vi "RobotMain.vi"() -> ()   [LabVIEW 2016]
uses:
  <vilib>/NXT/Subs/LVHSConnector.ctl
  <vilib>/NXT/LegoClasses/BrickReference/BrickReference.lvclass
  <vilib>/NXT/Subs/ColorSensorColors.ctl
  booleanos.ctl
  parametros.ctl
  <vilib>/NXT/Block Support/NXT_InputPort.ctl
  caracteristicas.ctl
  <vilib>/NXT/Block Support/NXT_ButtonSelector.ctl
  <vilib>/NXT/Block Support/NXT_OutputPort.ctl
  <vilib>/NXT/Dual Mode Library/Display/clearDisplay.vi
  <vilib>/NXT/NXTIO Xnodes/NXTIONodeSubVIs/NXTMoveMotors.vi
  <vilib>/NXT/Dual Mode Library/Sensors/readNXTButton.vi
  <vilib>/NXT/NXTIO Xnodes/NXTIONodeSubVIs/NXTStopMotors.vi
  <vilib>/NXT/Dual Mode Library/Waits/Wait_Btn_Press.vi
  <vilib>/NXT/NXTIO Xnodes/AddressXNode/NXTIOAddress.xnode
  <vilib>/NXT/NXTIO Xnodes/NXTIOXNode/NXTIO.xnode
panel:
  out "Boolean 5":bool=TRUE
  out "Boolean 4":bool
  out "Boolean 3":bool
  out "Boolean 2":bool
  out "Boolean":bool
  out "Ang_giroscopio":sgl
  in  "Movimentos \nStop":enum16{"Nada", "Front", "Pega", "Fim"}(ring)
  out "Enable\nreforço SM":bool
  out "Direction Bool":bool
  out "Booleanos e Contadores":T1={"Correct"=FALSE, "Enable State change"=TRUE, "First End"=FALSE, "Intersections crossed"=0.0, "Intersections crossed total"=0.0, "Bonecos"=0.0}
  out "Características":T2={"Colors and Directions"=[enum."Zero", enum."Zero", enum."Zero", enum."Zero", enum."Zero", enum."Zero"], "Direction"=enum."Right", "CS"=enum."Street", "Old Color"=enum."White"}
  in  "Características Iniciais":T2={"Colors and Directions"=[enum."Zero", enum."Zero", enum."Zero", enum."Zero", enum."Zero", enum."Zero"], "Direction"=enum."Right", "CS"=enum."Street", "Old Color"=enum."White"}
  out "Enable 2":bool
  out "Enable":bool
  in  "SC in":bool=TRUE
  in  "CS":T4(ring)
  in  "Parâmetros Iniciais":T5={"Gyro Port"=0, "Sensor - Left"=3, "Sensor - Right"=2, "     Color \nSensor Port"=1, "Kp Front"=0.5, "Motor speed"=-15, "Distance to street"=15.0, "Motor speed turns"=16, "Kp Curvas"=0.3} {"Kp Front" format="%.3f"; "Color \nSensor Port" items=["Port 1", "Port 2", "Port 3", "Port 4"]; "Sensor - Right" items=["Port 1", "Port 2", "Port 3", "Port 4"]; "Sensor - Left" items=["Port 1", "Port 2", "Port 3", "Port 4"]; "Gyro Port" items=["Port 1", "Port 2", "Port 3", "Port 4"]}
  in  "Booleanos e Contadores Iniciais":T1={"Correct"=FALSE, "Enable State change"=TRUE, "First End"=FALSE, "Intersections crossed"=0.0, "Intersections crossed total"=0.0, "Bonecos"=0.0} caption="Booleanos e Contadores"
  out "IdentifyCollor":T3=enum."White"
  out "Collor":T3
  out "NXT/EV3 2":T7
  in  "NXT/EV3":T7
  # "Permite que ocorra troca \nde estados se True e interrompe-as \nse False."
  # "Booleano que retorna F quando chega em Delivery.\nGarantindo que não contará\nmais intersections"
  # "Salva o total de interseções \ncruzadas"
  # "Contador de quantas \ninterseções foram cruzadas.\nSoma ao acertar"
  # "black"
  # "blue"
  # "green"
  # "yellow"
  # "red"
  # "black"
  # "blue"
  # "green"
  # "yellow"
  # "red"
  # "Permite que ocorra troca \nde estados se True e interrompe-as \nse False."
  # "Booleano que retorna F quando chega em Delivery.\nGarantindo que não contará\nmais intersections"
  # "Salva o total de interseções \ncruzadas"
  # "Contador de quantas \ninterseções foram cruzadas.\nSoma ao acertar"
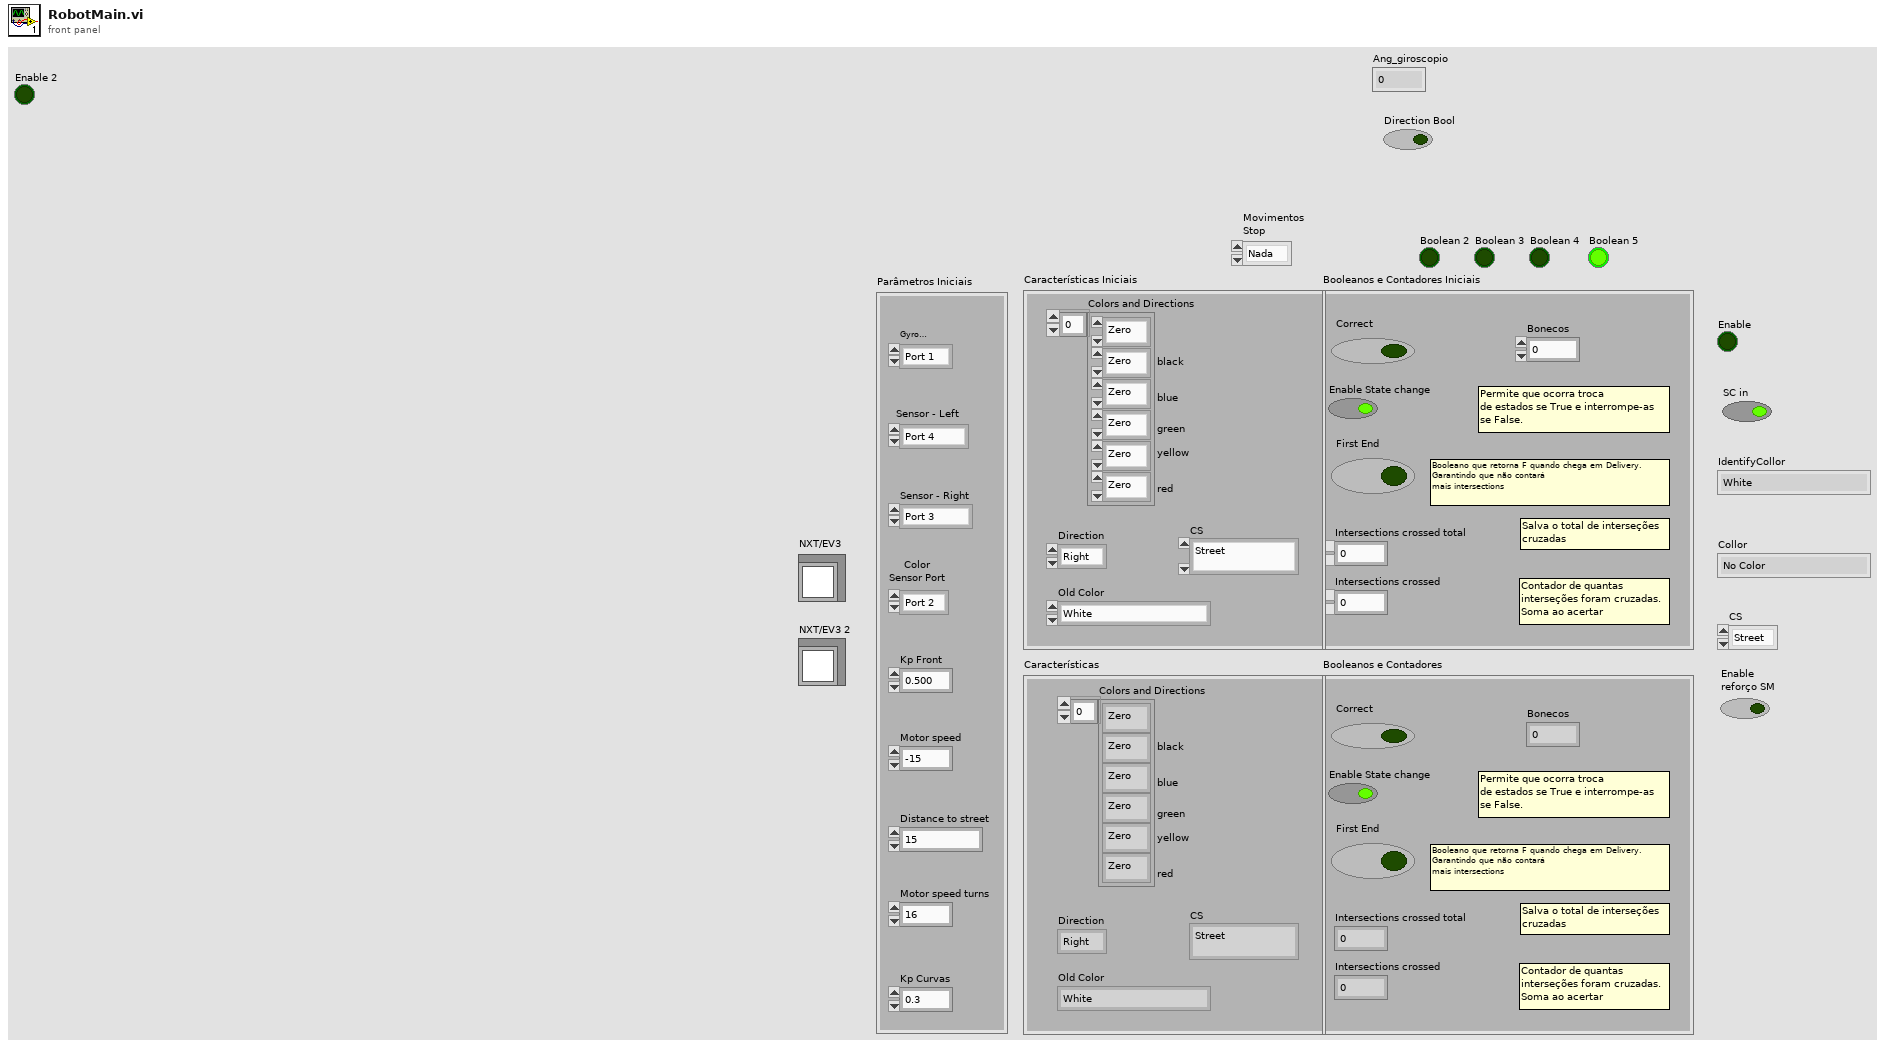
[diagram p1: front panel]
types:
  T1 = typedef "booleanos.ctl" = cluster{"Correct":bool, "Enable State change":bool, "First End":bool, "Intersections crossed":dbl, "Intersections crossed total":dbl, "Bonecos":dbl}
  T2 = typedef "caracteristicas.ctl" = cluster{"Colors and Directions":enum16{"Zero", "Right", "Front", "Left"}[], "Direction":enum16{"Zero", "Right", "Front", "Left"}, "CS":enum16{"Street", "Intersection", "End", "Stop", "Square", "Delivery", "Empty"}, "Old Color":T3}
  T3 = typedef "ColorSensorColors.ctl" = enum16{"No Color", "Black", "Blue", "Green", "Yellow", "Red", "White", "Brown"}
  T4 = enum16{"Street", "Intersection", "End", "Stop", "Square", "Delivery"}
  T5 = typedef "parametros.ctl" = cluster{"Gyro Port":T6, "Sensor - Left":T6, "Sensor - Right":T6, "     Color \nSensor Port":T6, "Kp Front":dbl, "Motor speed":i32, "Distance to street":dbl, "Motor speed turns":i32, "Kp Curvas":dbl}
  T6 = typedef "NXT_InputPort.ctl" = u32
  T7 = typedef "LVHSConnector.ctl" = refnum<class "BrickReference.lvclass">
  T8 = typedef "NXT_OutputPort.ctl" = u8
  T9 = enum16{"Street", "Intersection", "End", "Stop", "Square", "Delivery", "Empty"}
  T10 = typedef "NXT_ButtonSelector.ctl" = u16
  T11 = cluster{"Colors and Directions":enum16{"Zero", "Right", "Front", "Left"}[], "Direction":enum16{"Zero", "Right", "Front", "Left"}, "CS":enum16{"Street", "Intersection", "End", "Stop", "Square", "Delivery"}, "Old Color":T3}
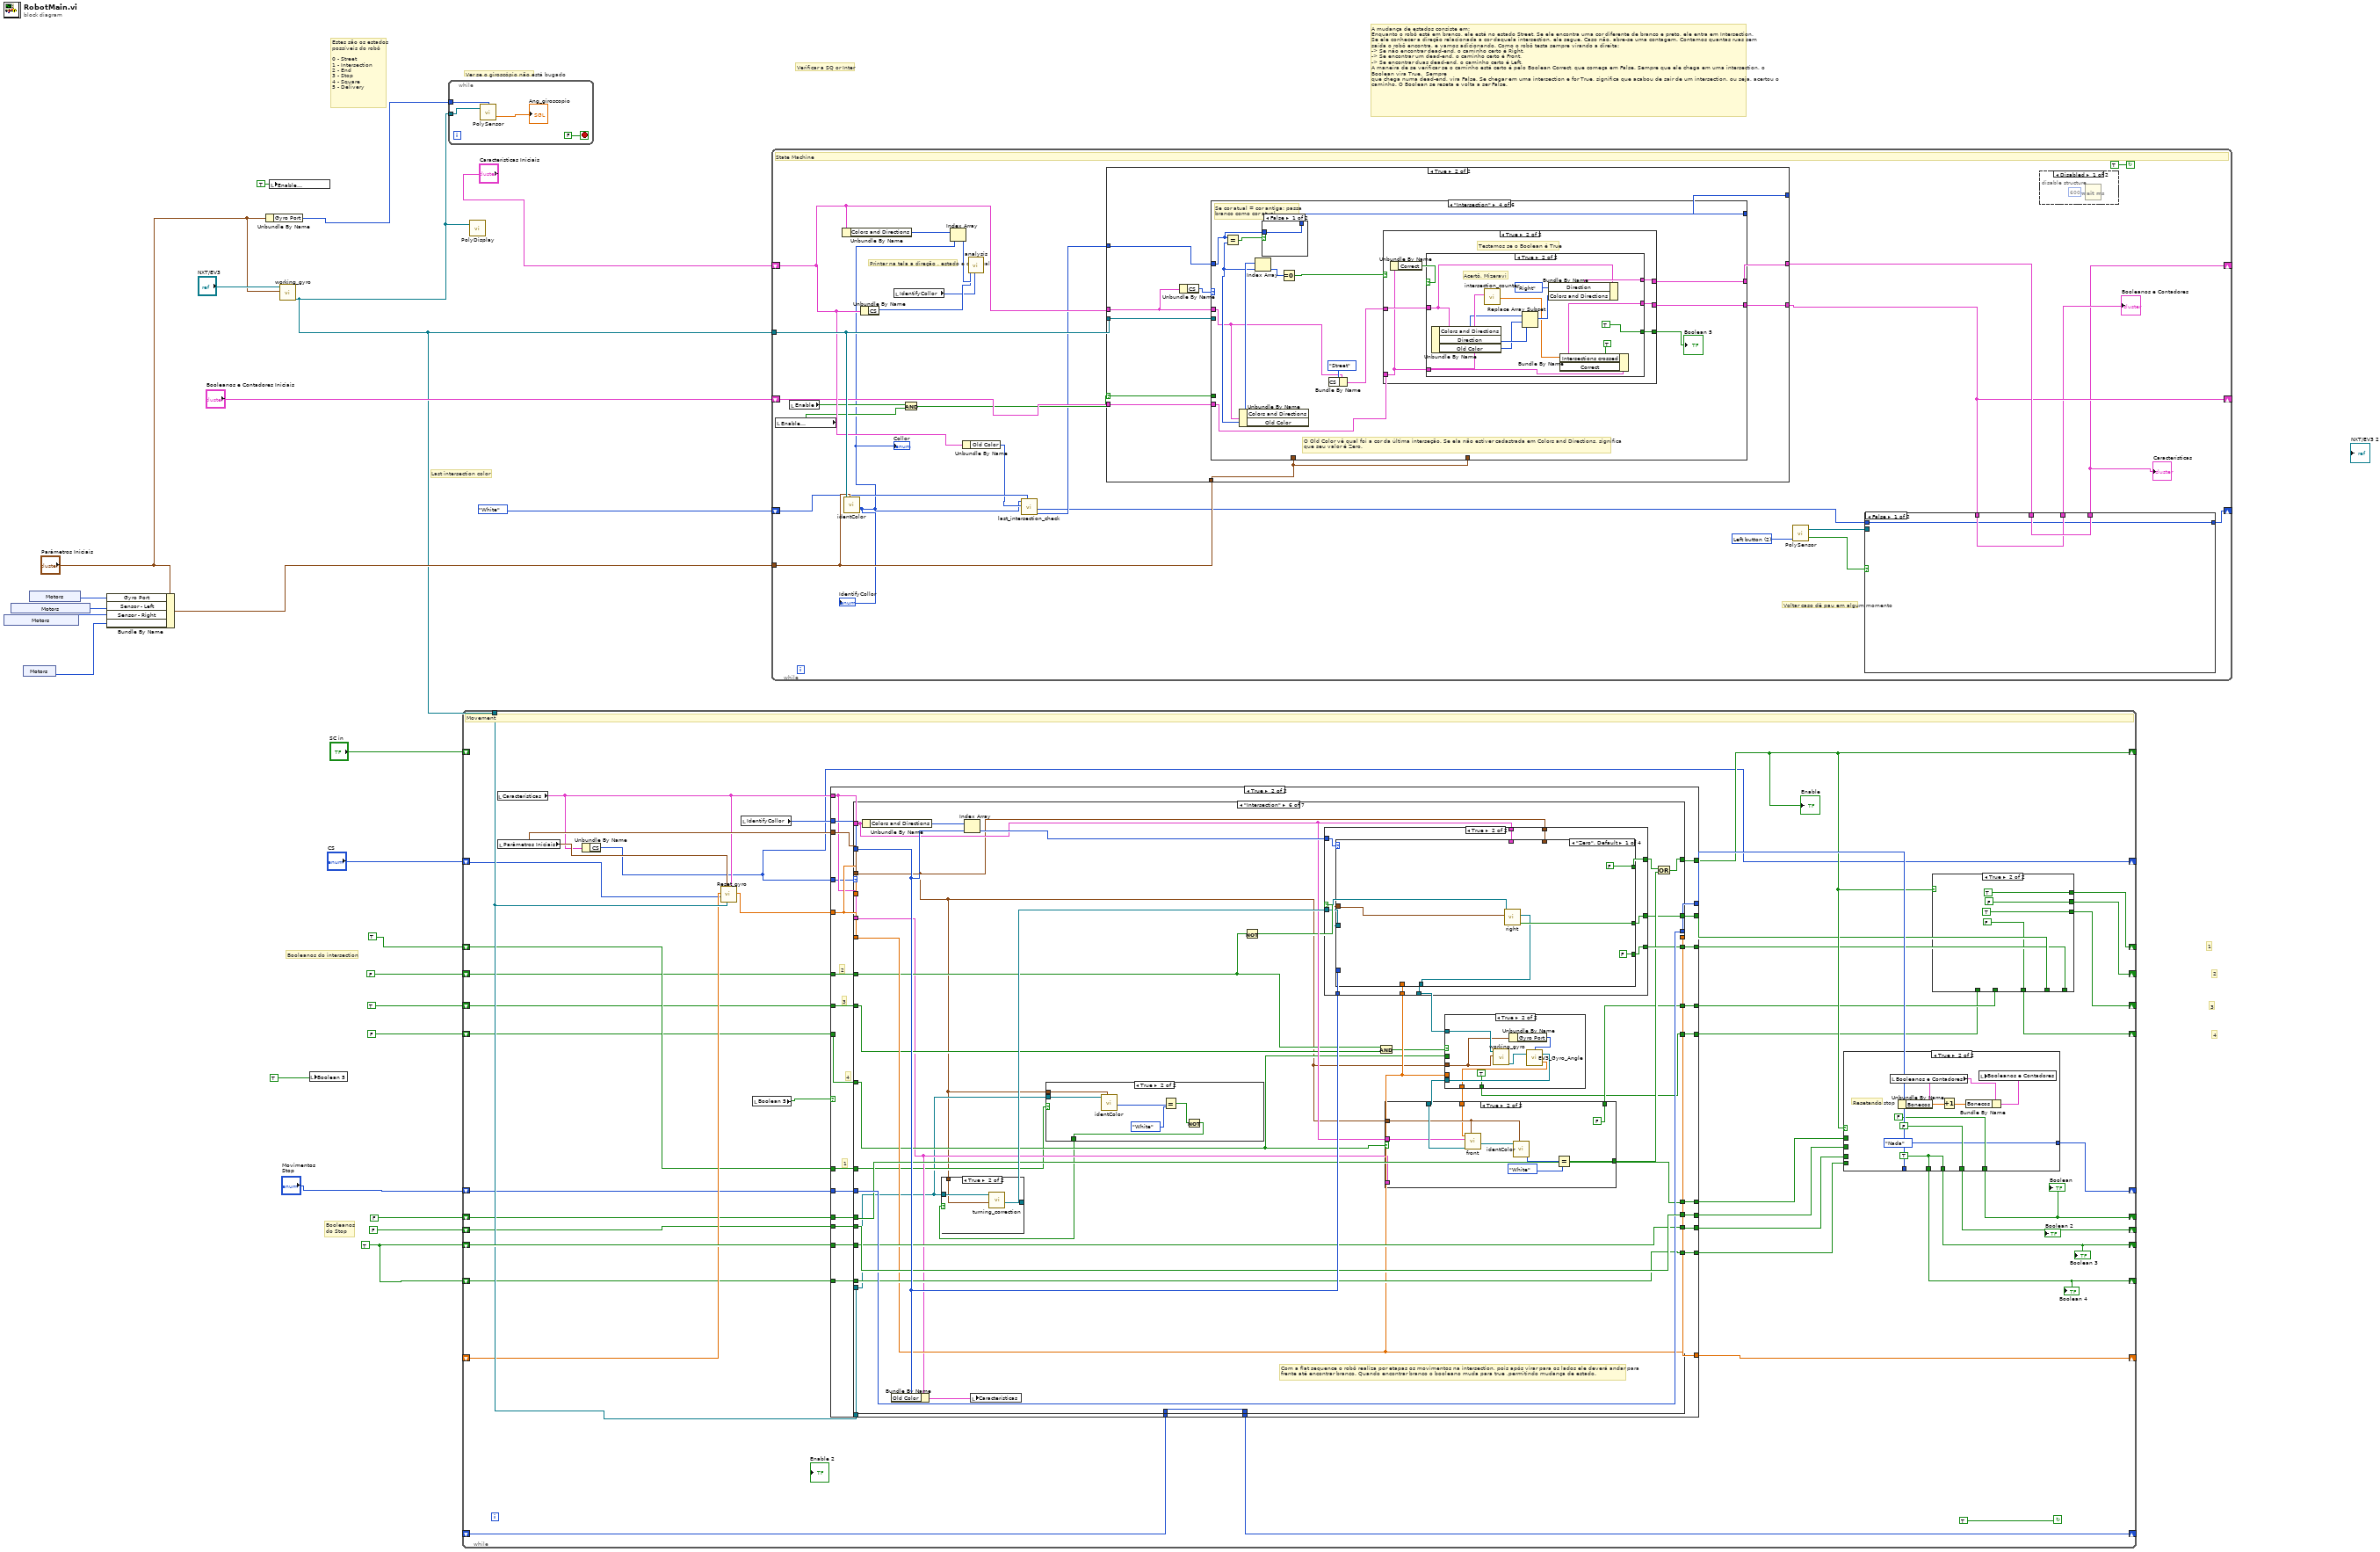
[diagram p0: block diagram]
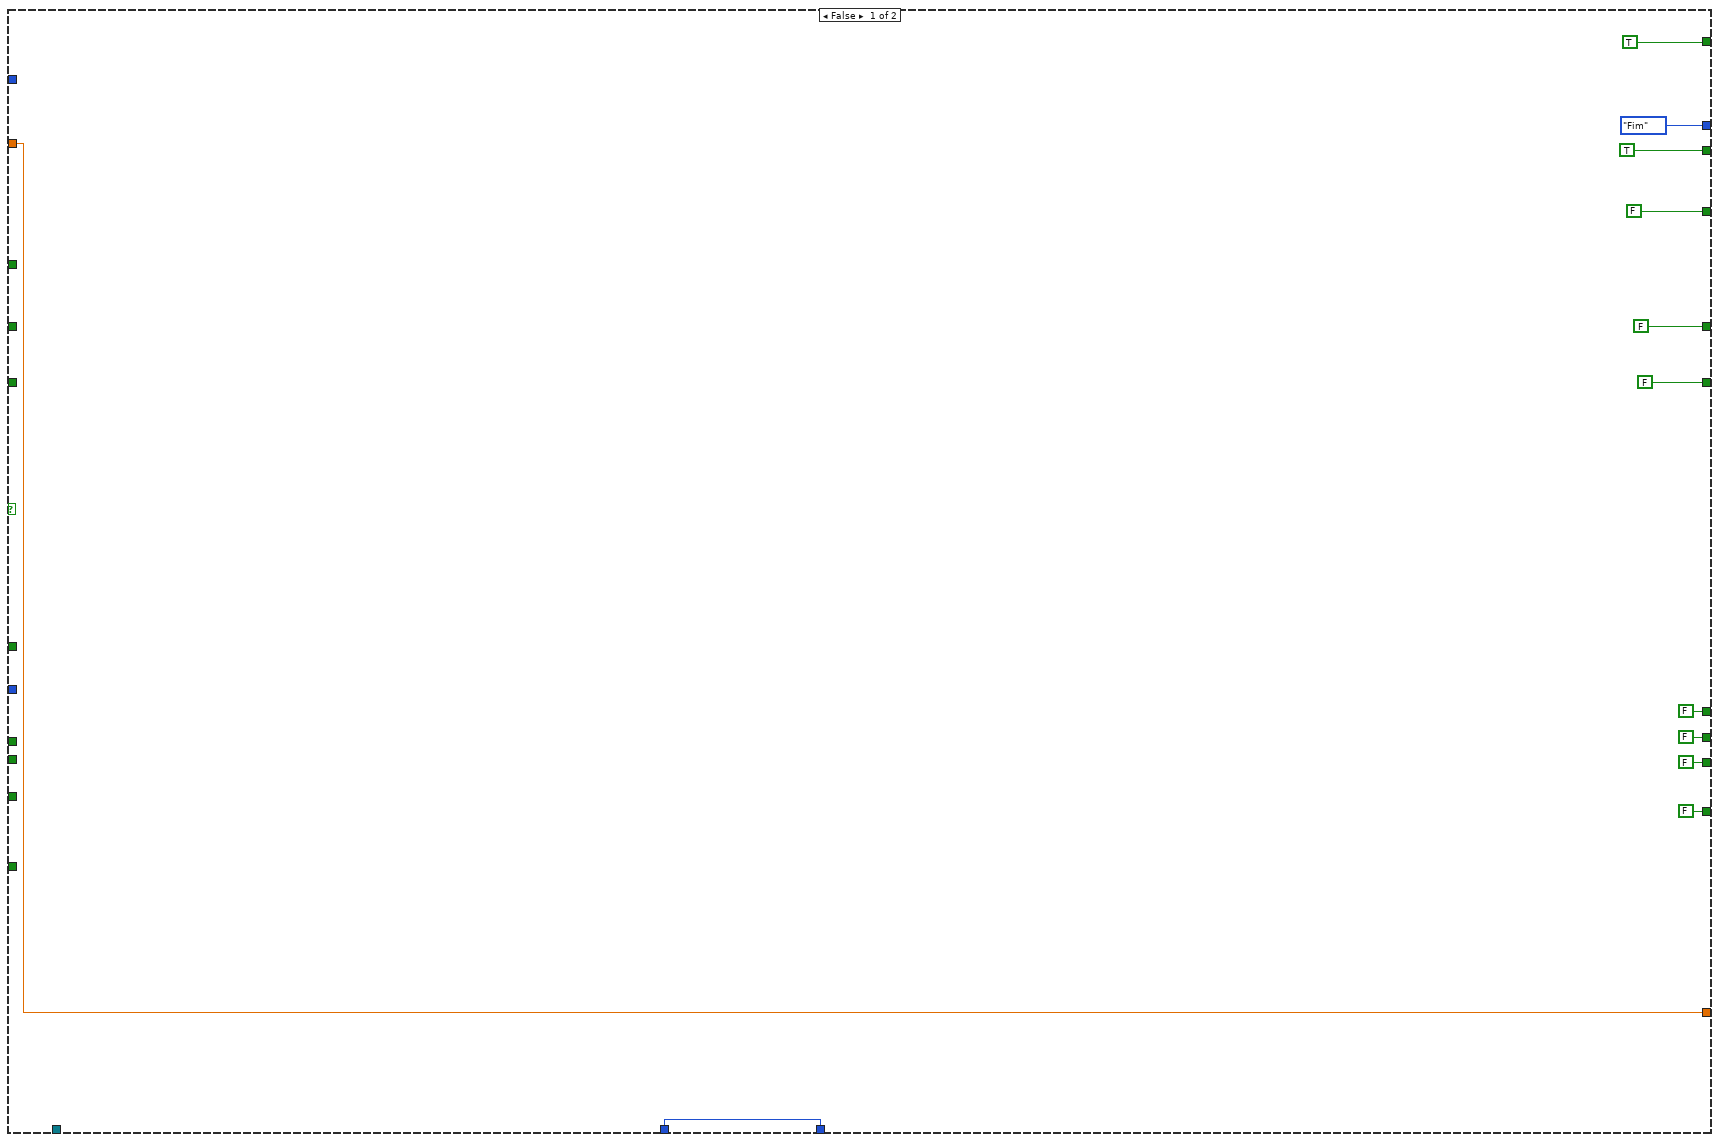
[diagram p2: hidden frame]
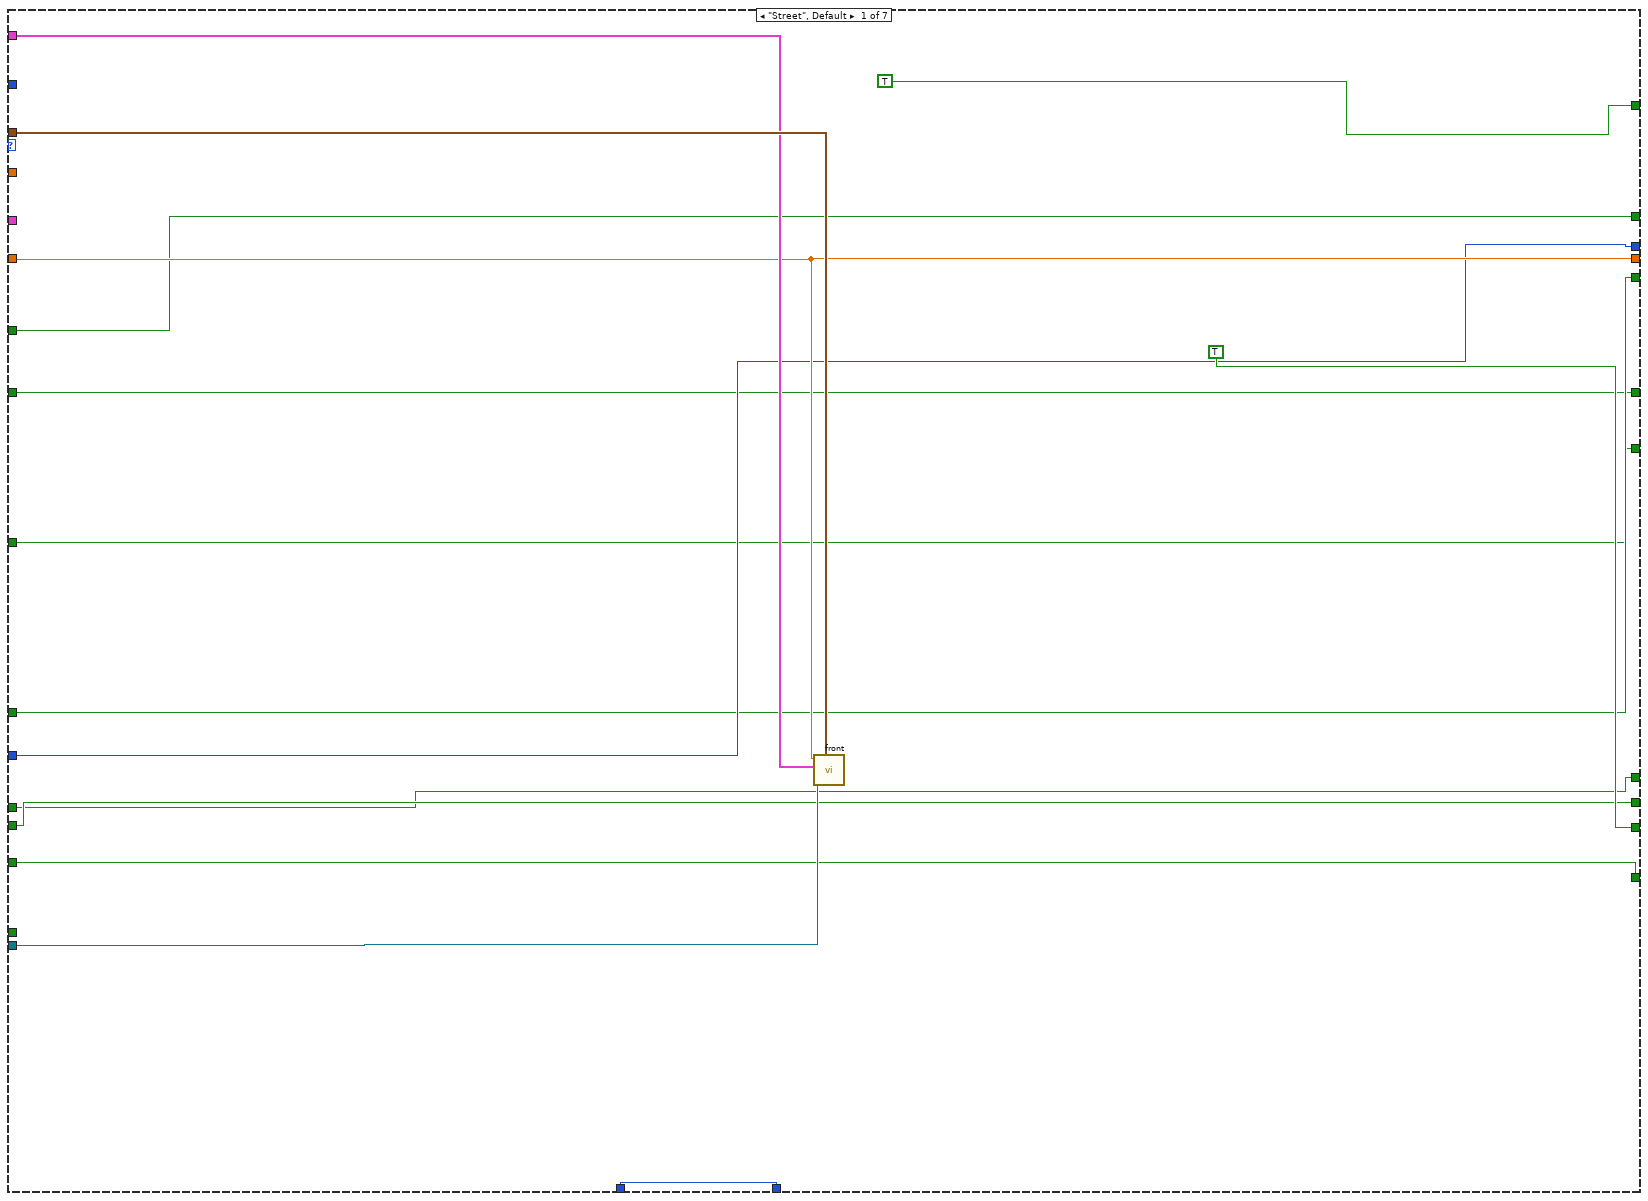
[diagram p3: hidden frame]
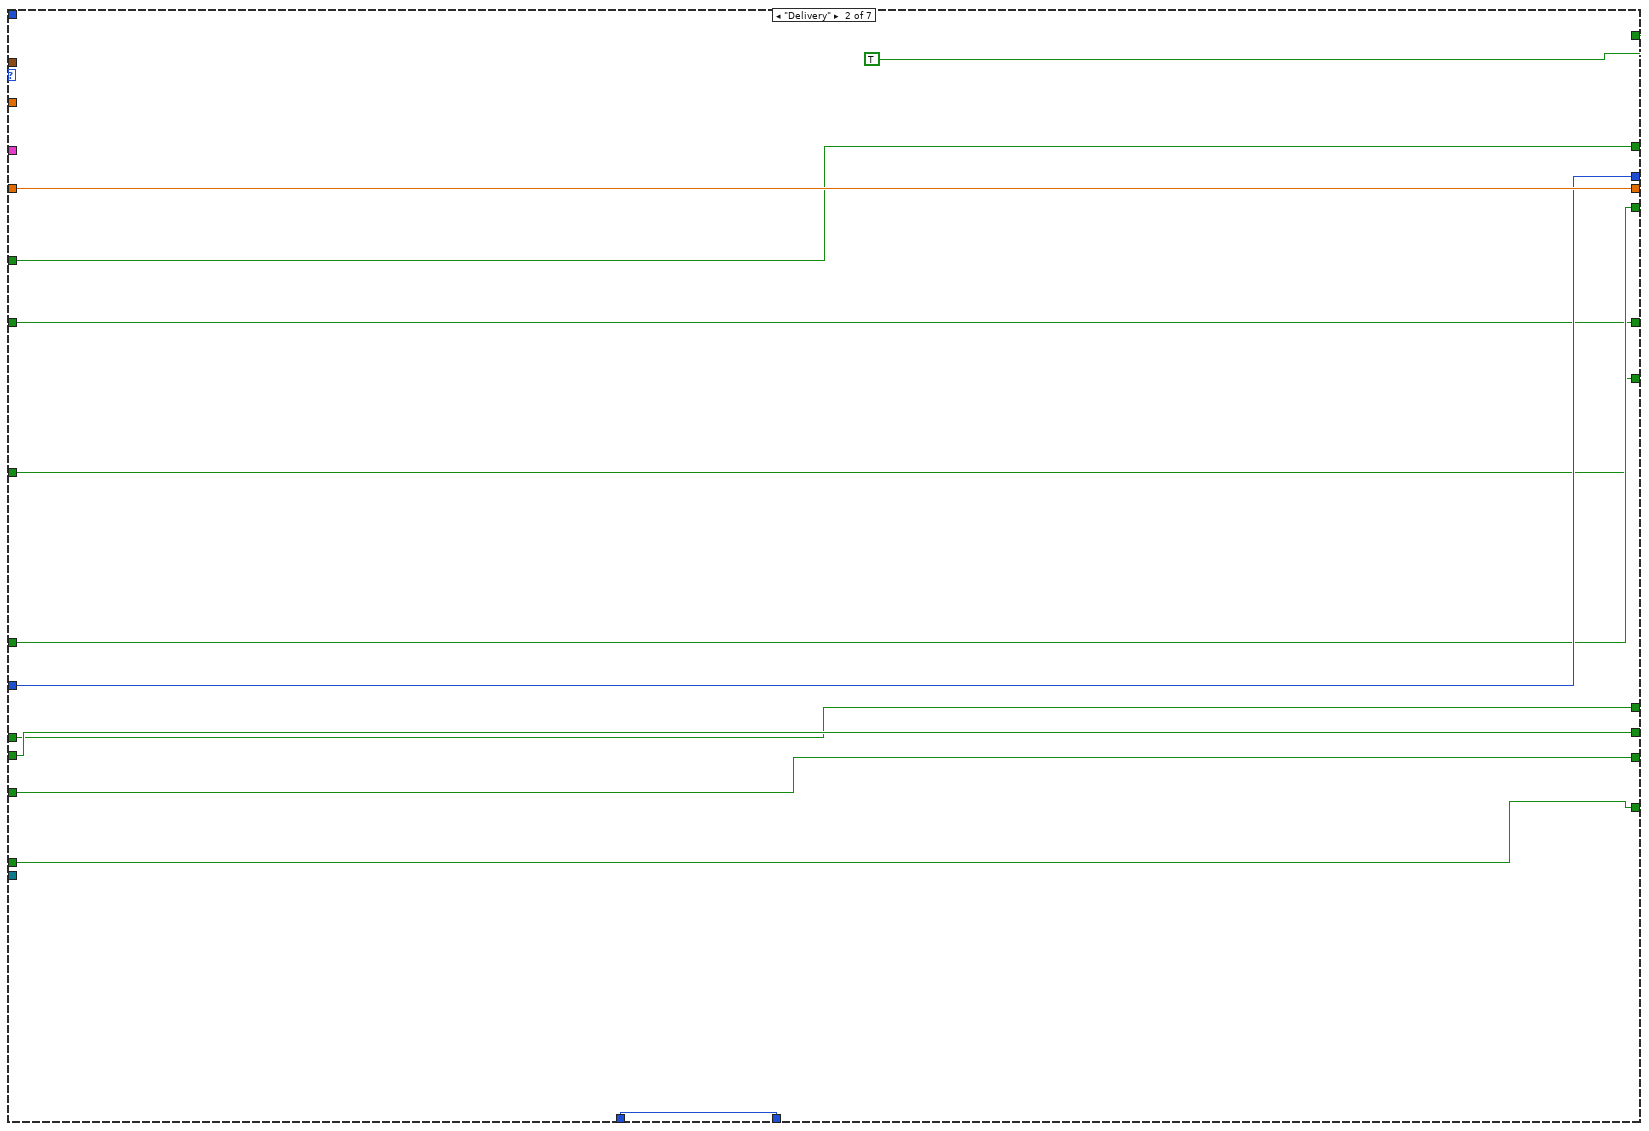
[diagram p4: hidden frame]
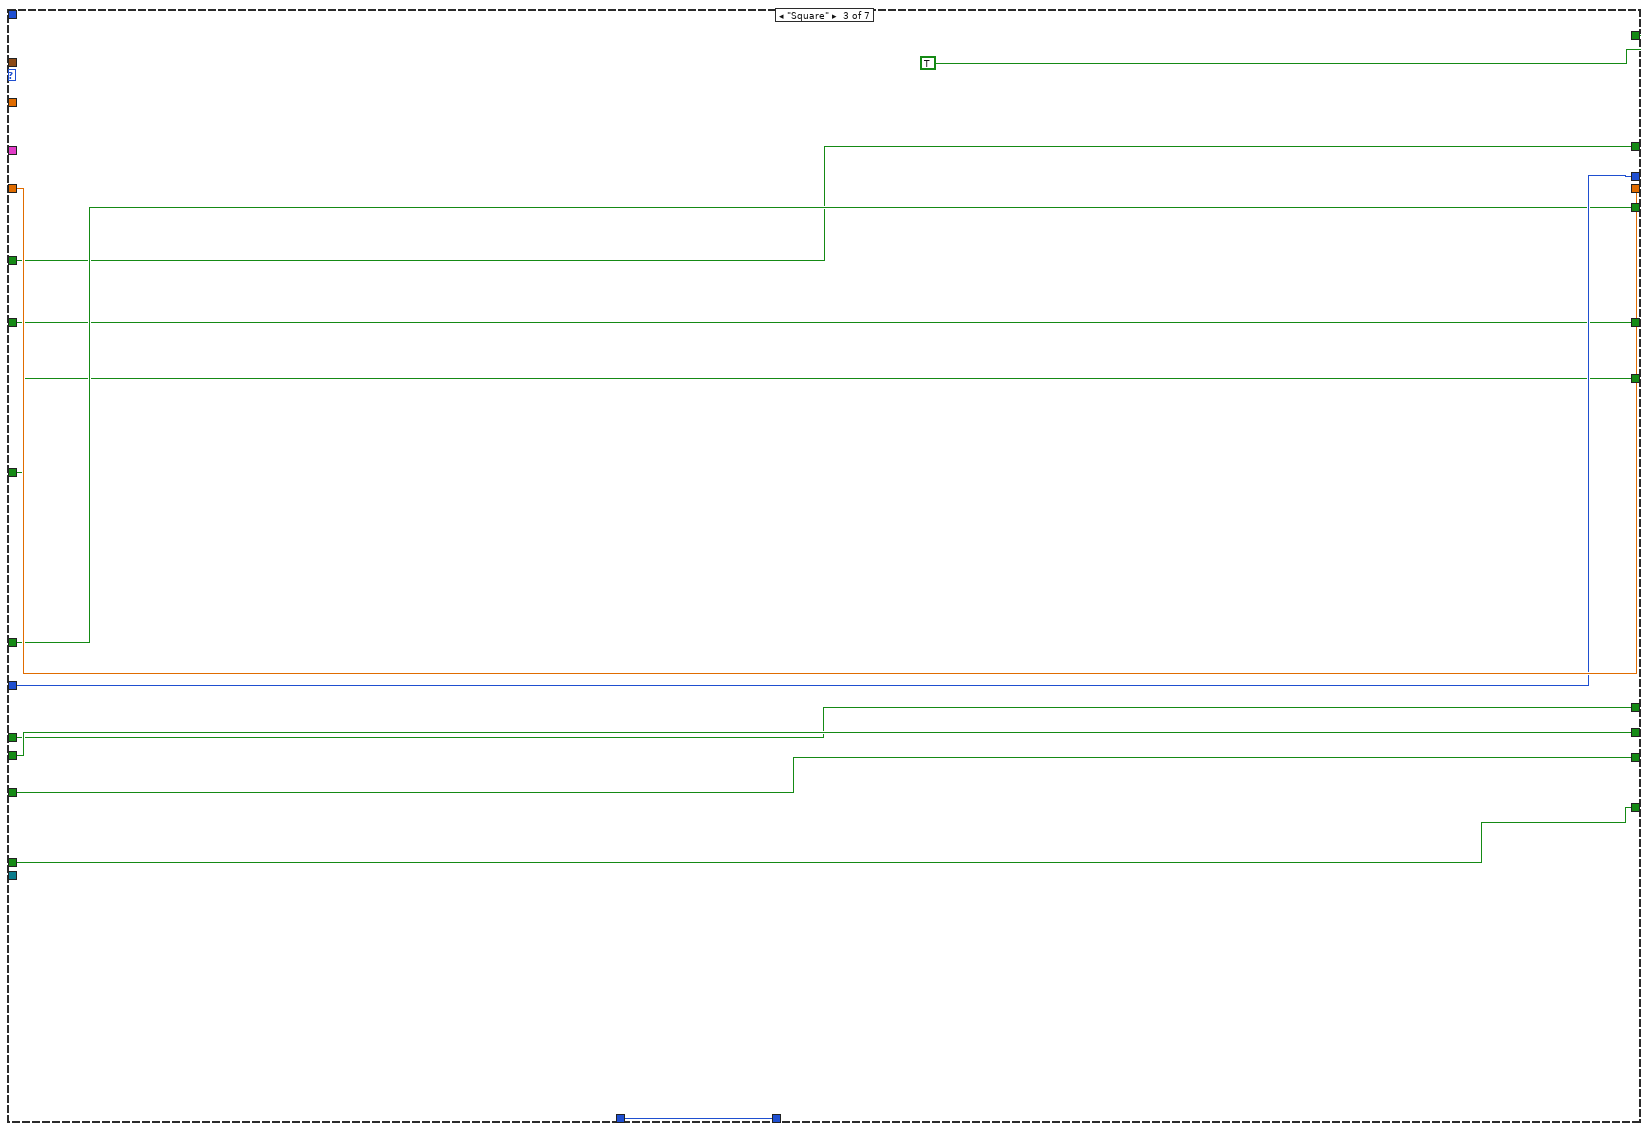
[diagram p5: hidden frame]
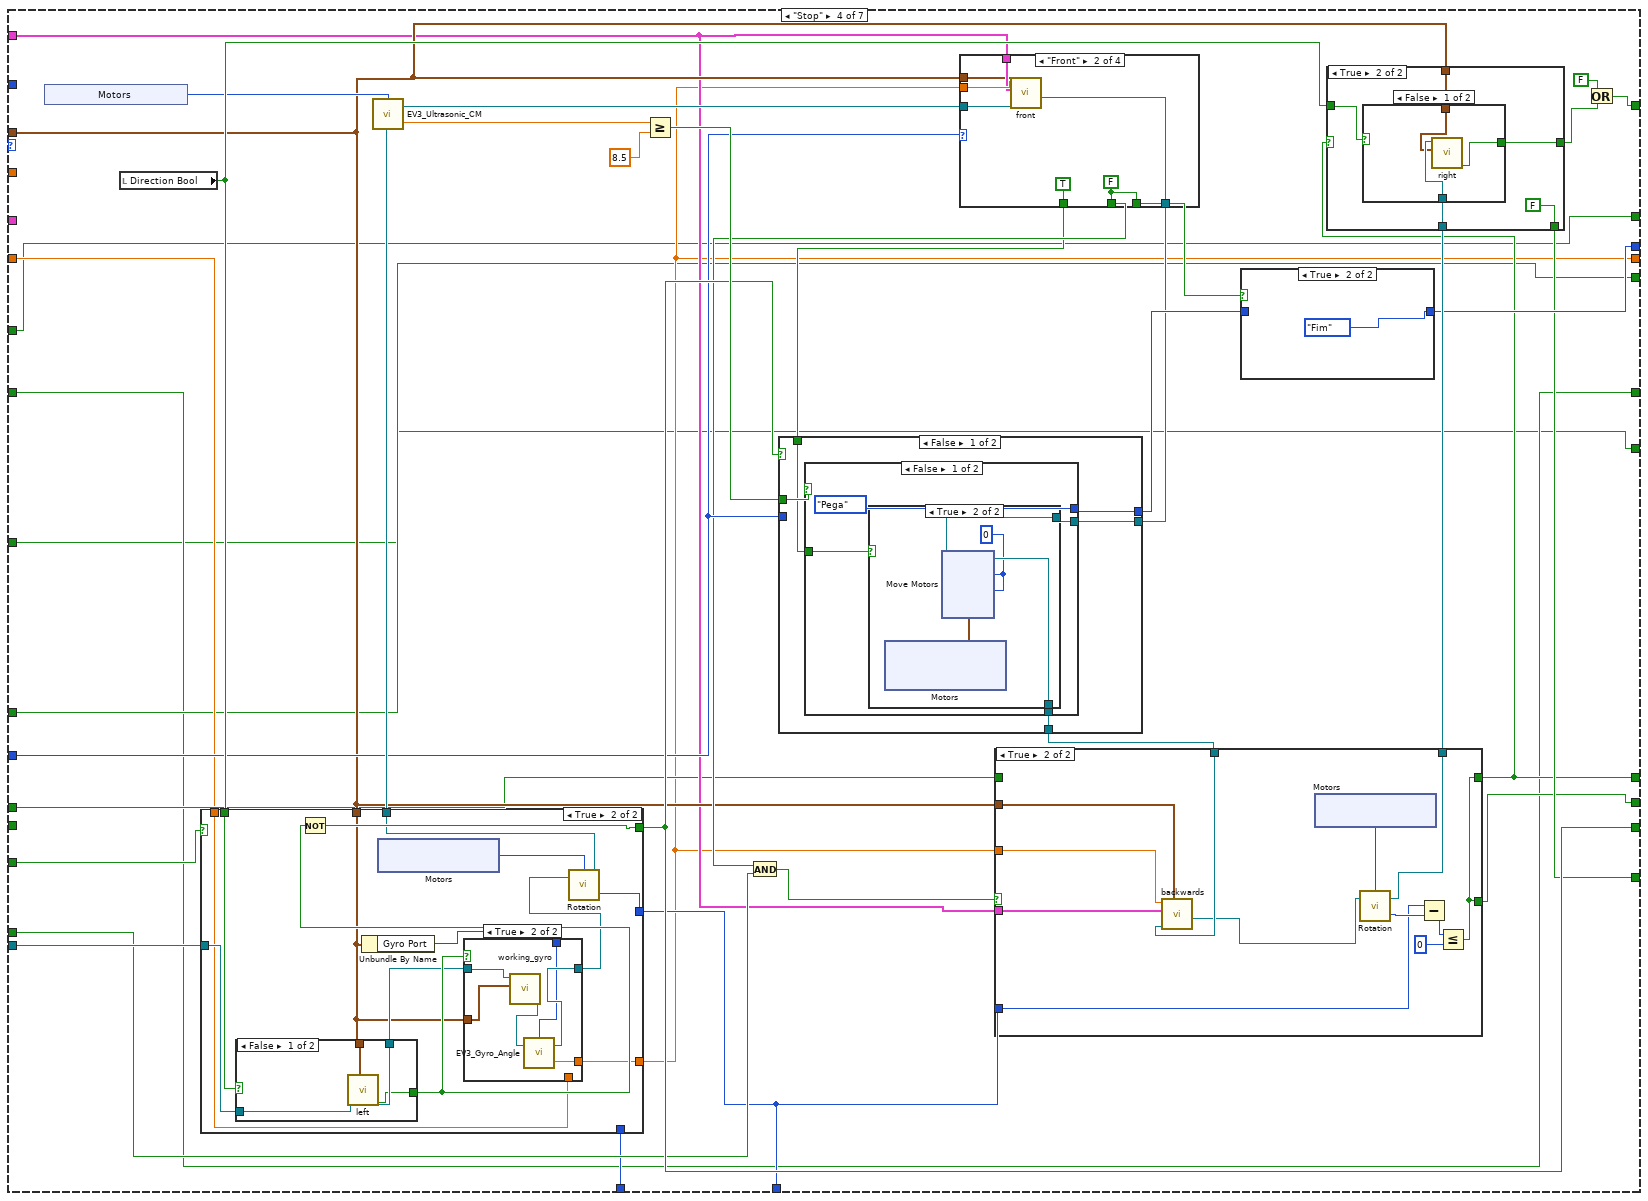
[diagram p6: hidden frame]
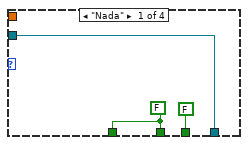
[diagram p7: hidden frame]
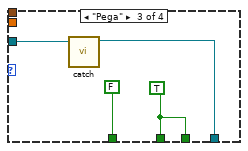
[diagram p8: hidden frame]
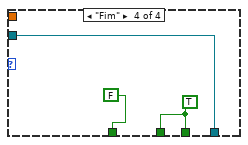
[diagram p9: hidden frame]
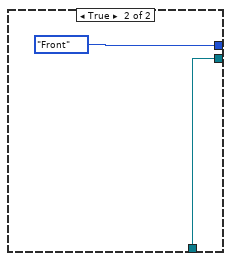
[diagram p12: hidden frame]
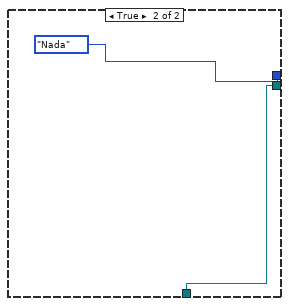
[diagram p13: hidden frame]
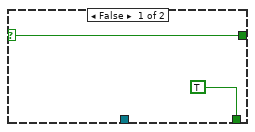
[diagram p14: hidden frame]
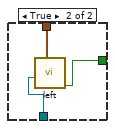
[diagram p15: hidden frame]
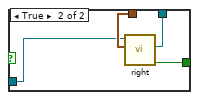
[diagram p19: hidden frame]
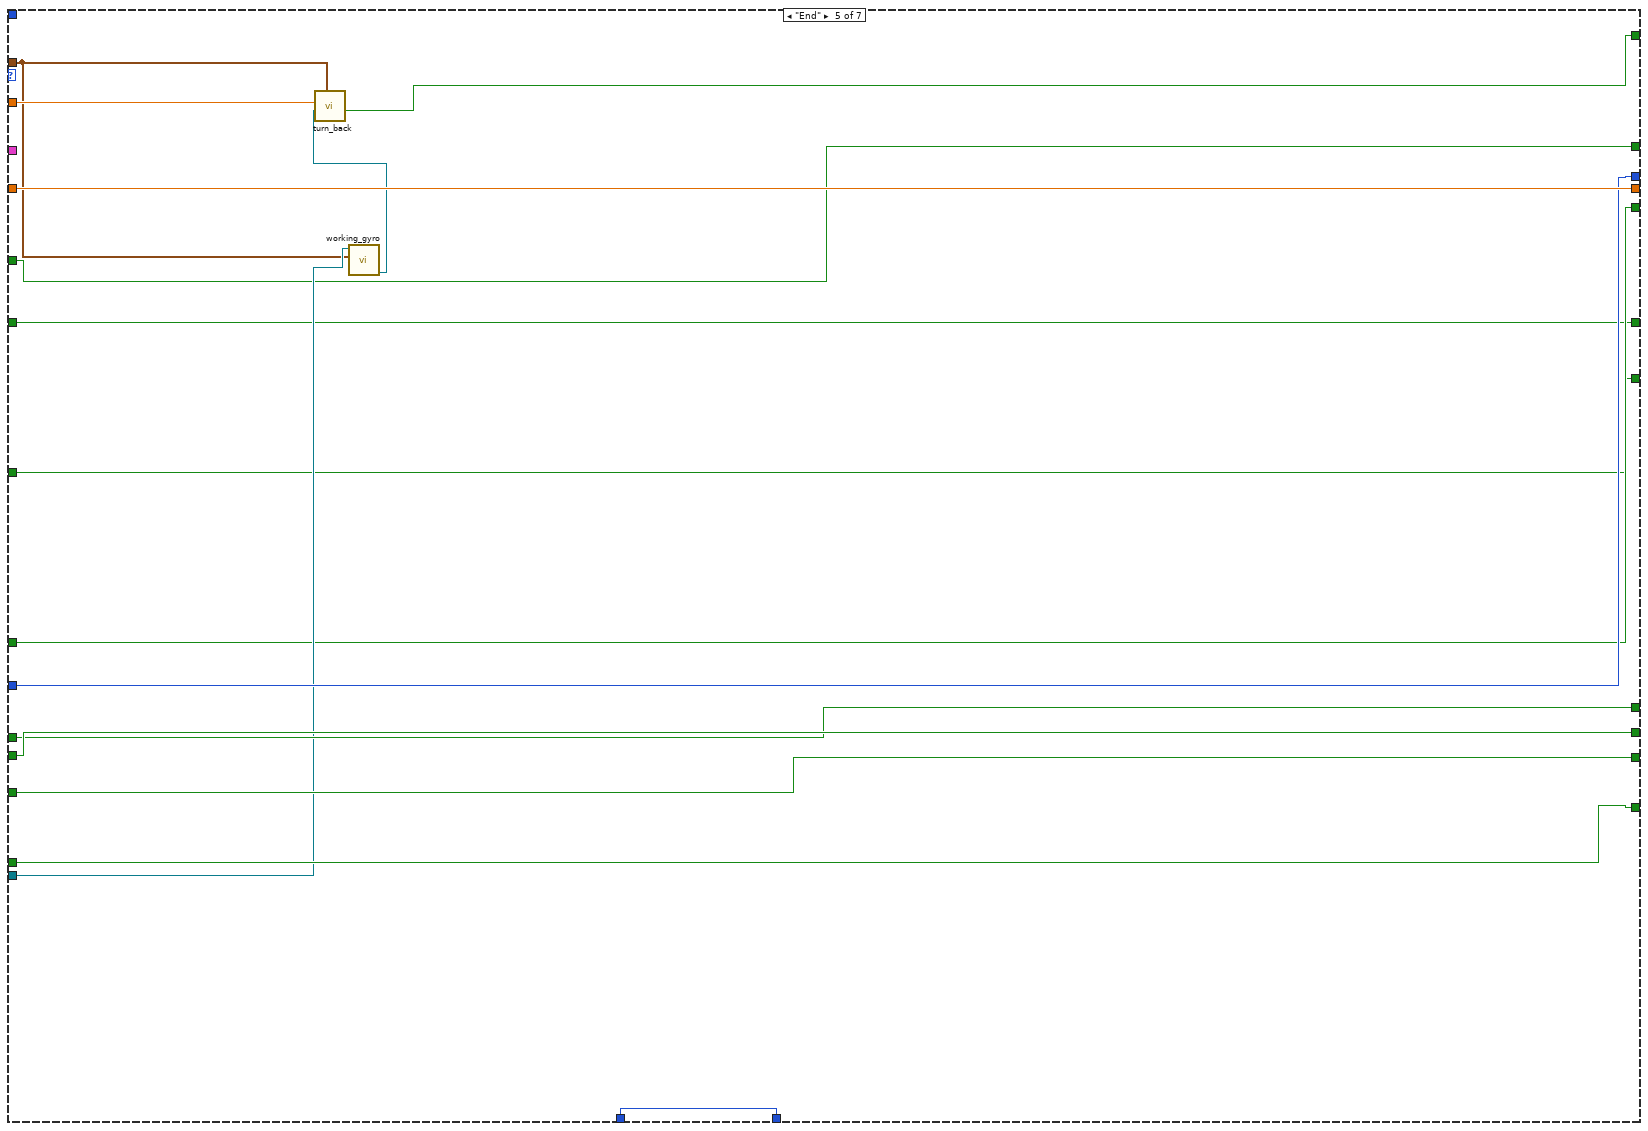
[diagram p20: hidden frame]
diagram:
  w13 = TRUE
  # "4"
  # "1"
  # "2"
  # "3"
  # "Booleanos do intersection"
  # "Booleanos\ndo Stop"
  # "Ver se o giroscópio não está bugado"
  # "Last intersection color"
  # "Verificar a SQ or Inter"
  # "A mudança de estados consiste em:\nEnquanto o robô está em branco, ele está no estado Street. Se ele encontra uma cor diferente de branco e preto, ele entra em Intersection.\nSe ele conhecer a direção relacionada a cor daquela intersection, ele segue. Caso não, abre-se uma contagem. Contamos quantas ruas sem \nsaída o robô encontra, e vamos adicionando. Como o robô testa sempre virando a direita:\n-> Se não encontrar dead-end, o caminho certo é Right.\n-> Se encontrar um dead-end, o caminho certo é Front.\n-> Se encontrar duas dead-end, o caminho certo é Left.\nA maneira de se verificar se o caminho está certo é pelo Boolean Correct, que começa em False. Sempre que ele chega em uma intersection, o Boolean vira True.  Sempre\nque chega numa dead-end, vira False. Se chegar em uma intersection e for True, significa que acabou de sair de um intersection, ou seja, acertou o\ncaminho. O Boolean se reseta e volta a ser False."
  # "Estes são os estados\npossíveis do robô\n\n0 - Street\n1 - Intersection\n2 - End\n3 - Stop\n4 - Square\n5 - Delivery"
  n1 = xnode "Motors"() -> ("Sensor"=w20:T6)
  n2 = xnode "Motors"() -> ("Sensor"=w21:T6)
  n3 = xnode "Motors"() -> ("Sensor"=w19:T6)
  n4 = xnode "Motors"() -> ("Sensor"=w22:T6)
  n5 = Bundle By Name(cluster="Parâmetros Iniciais", "Gyro Port"=w22, "Sensor - Left"=w21, "Sensor - Right"=w20, "Color \nSensor Port"=w19) -> (w23:T5)
  n6 = Unbundle By Name("Parâmetros Iniciais") -> ("Gyro Port"=w9:T6)
  n7 = local write "Enable\nreforço SM"(TRUE ("Enable\nreforço SM")) -> ()
  n8 = call "working_gyro.vi"("Parâmetros Iniciais"="Parâmetros Iniciais", "NXT/EV3"="NXT/EV3") -> ("NXT/EV3 2"=w7:T7)  [unwired: 9 in]
  n9 = local write "Boolean 5"(TRUE) -> ()
  n10 = while {
    tunnel: w7 -> [w28]
    tunnel: w9 -> [w27]
    stop <- FALSE stop-if-true
    n11 = call-poly <vilib>:"PolySensor.vi"("NXT/EV3"=w28, "Port (Port 1)"=w27) -> ("Degrees"=→"Ang_giroscopio":sgl)  [unwired: 1 in, 1 out]
  }
  n12 = while {
    shift-right: [w67] -> _
    shift-left: _ -> [w63]
    shift-right: [w31] -> _
    shift-left: "CS" -> [w33]
    tunnel: w7 -> [w65]
    shift-right: [w44] -> _
    shift-left: "SC in" -> [_]
    shift-right: [w49] -> _
    shift-left: w13 -> [w66]
    shift-right: [w50] -> _
    shift-left: FALSE ("Boolean") -> [w61]
    shift-right: [w47] -> _
    shift-left: "Movimentos \nStop" -> [w60]
    shift-right: [w48] -> _
    shift-left: w13 -> [w59]
    shift-right: [w58] -> _
    shift-left: _ -> [w57]
    shift-right: [w51] -> _
    shift-left: FALSE ("Boolean") -> [w56]
    shift-right: [w43] -> _
    shift-left: TRUE -> [w45]
    shift-right: [w42] -> _
    shift-left: FALSE -> [w32]
    shift-right: [w39] -> _
    shift-left: TRUE -> [w41]
    shift-right: [w37] -> _
    shift-left: FALSE -> [w40]
    stop <- TRUE continue-if-true
    # "Movement"
    n13 = local read "Características"() -> (w34:T2)
    n14 = local read "Parâmetros Iniciais"() -> (w64:T5)
    n15 = Unbundle By Name(w34) -> ("CS"=w31:T9)
    n16 = call "Reset_gyro.vi"("Características Iniciais"=w34, "NXT/EV3"=w65, "Parâmetros Iniciais"=w64, "CS"=w33, "First Angle IN"=w63) -> ("First Angle OUT"=w62:sgl)  [unwired: 6 in]
    n17 = local read "IdentifyCollor"() -> (w69:T3)
    n18 = local read "Boolean 5"() -> (w29:bool)
    n19 = case shown="True" w29 {
      tunnel: w69 -> [_ w109]
      tunnel: [w79 w108] -> w67
      tunnel: w66 -> [_ w107]
      tunnel: w65 -> [_ w106]
      tunnel: w64 -> [_ w105]
      tunnel: w62 -> [w79 w104]
      tunnel: w61 -> [_ w103]
      tunnel: w60 -> [_ w102]
      tunnel: w59 -> [_ w101]
      tunnel: [w70 w100] -> w58
      tunnel: w57 -> [w70 w99]
      tunnel: w56 -> [_ w98]
      tunnel: [FALSE ("Boolean") w97] -> w55
      tunnel: [FALSE ("Boolean") w96] -> w54
      tunnel: [FALSE w95] -> w53
      tunnel: [FALSE w94] -> w52
      tunnel: [enum16{"Nada", "Front", "Pega", "Fim"}."Fim" ("Movimentos \nStop") w93] -> w46
      tunnel: w45 -> [_ w92]
      tunnel: [TRUE w91] -> w44
      tunnel: w41 -> [_ w90]
      tunnel: w40 -> [_ w89]
      tunnel: [FALSE w88] -> w38
      tunnel: [FALSE w87] -> w36
      tunnel: [TRUE ("x = y?") w86] -> w35
      tunnel: w34 -> [_ w85]
      tunnel: w32 -> [_ w84]
      tunnel: w31 -> [_ w83]
      tunnel: [FALSE w82] -> w30
      frame False {
      }
      frame True {
        # "4"
        # "1"
        # "2"
        # "3"
        n20 = case shown="\"Intersection\"" w83 {
          tunnel: [TRUE TRUE ("x = y?") TRUE ("x = y?") w165 w311 w331 TRUE] -> w91
          tunnel: w106 -> [w124 _ _ w185 w303 w315 _]
          tunnel: w109 -> [_ _ _ _ _ w342 _]
          tunnel: w105 -> [w123 _ _ w160 w301 w314 _]
          tunnel: w85 -> [w122 _ _ w159 _ w333 _]
          tunnel: w104 -> [w121 w135 w147 w153 w312 w325 w429]
          tunnel: [w121 w135 w147 w154 w312 w325 w429] -> w108
          tunnel: w85 -> [_ _ _ _ _ w317 _]
          tunnel: w104 -> [_ _ _ _ w310 _ _]
          tunnel: w107 -> [w116 w134 w146 w186 w309 w335 w425]
          tunnel: [TRUE w134 w146 w173 w309 w335 TRUE] -> w95
          tunnel: [w118 w133 w145 w157 w308 w340 w427] -> w96
          tunnel: w103 -> [w118 w133 w145 _ w308 w340 w427]
          tunnel: w102 -> [w117 w132 w144 w172 w307 w339 w430]
          tunnel: [w117 w132 w144 w175 w307 w339 w430] -> w93
          tunnel: [w116 w131 w143 w169 w306 w338 w425] -> w94
          tunnel: w101 -> [_ w131 w143 w168 w306 w338 _]
          tunnel: [w115 w130 w142 w167 w305 w337 w424] -> w100
          tunnel: w99 -> [w115 w130 w142 w166 w305 w337 w424]
          tunnel: [w114 w129 w141 w155 w304 w334 w428] -> w97
          tunnel: w98 -> [w114 w129 w141 w156 w304 w334 w428]
          tunnel: w92 -> [w113 w128 w140 w152 w300 w316 w423]
          tunnel: [w113 w128 w140 w152 w300 w336 w423] -> w82
          tunnel: w84 -> [w110 w125 w137 w149 w297 w324 w420]
          tunnel: w90 -> [w112 w127 w139 w151 w299 w322 w422]
          tunnel: [w112 w127 w139 w151 w299 w321 w422] -> w88
          tunnel: w89 -> [w111 w126 w138 w150 w298 w318 w421]
          tunnel: [w111 w126 w138 w150 w298 w320 w421] -> w87
          tunnel: [w110 w125 w137 w149 w297 w319 w420] -> w86
          frame "Street", Default {
            n21 = call "front.vi"("Parâmetros Ini 2"=w123, "NXT/EV3"=w124, "Características Ini"=w122, "First Angle"=w121) -> ()  [unwired: 7 in, 1 out]
          }
          frame "Delivery" {
          }
          frame "Square" {
          }
          frame "Stop" {
            n22 = xnode "Motors"() -> ("Sensor"=w164:T6)
            n23 = local read "Direction Bool"() -> (w180:bool)
            n24 = case shown="True" w186 {
              selector: w186 -> [w266 _]
              tunnel: w180 -> [_ w279]
              tunnel: [w266 w277] -> w173
              tunnel: w160 -> [_ w270]
              tunnel: w185 -> [w265 w278]
              tunnel: [w265 w275] -> w184
              tunnel: [w264 w274] -> w167
              tunnel: w166 -> [w264 _]
              tunnel: [w263 w268] -> w154
              tunnel: w153 -> [w263 w267]
              frame False {
              }
              frame True {
                n25 = case shown="False" w279 {
                  tunnel: w270 -> [w292 w296]
                  tunnel: w278 -> [w291 w295]
                  tunnel: [w290 w294] -> w272
                  tunnel: [w289 w293] -> w273
                  frame False {
                    n26 = call "left.vi"("Parâmetros Ini 2"=w292, "NXT/EV3"=w291) -> ("x = y?"=w289:bool, "NXT/EV3 2"=w290:T7)  [unwired: 8 in]
                  }
                  frame True {
                    n27 = call "right.vi"("Parâmetros Ini 2"=w296, "NXT/EV3"=w295) -> ("x = y?"=w293:bool, "NXT/EV3 2"=w294:T7)  [unwired: 8 in]
                  }
                }
                n28 = Not(x=w273) -> (.not. x?=w277:bool)
                n29 = Unbundle By Name(w270) -> ("Gyro Port"=w269:T6)
                n30 = xnode "Motors"() -> ("Motor"=w276:T8)
                n31 = case shown="True" w273 {
                  tunnel: w272 -> [w281 w287]
                  tunnel: [w281 w284] -> w271
                  tunnel: w270 -> [_ w286]
                  tunnel: w269 -> [_ w283]
                  tunnel: [w280 w282] -> w268
                  tunnel: w267 -> [w280 _]
                  frame False {
                  }
                  frame True {
                    n32 = call "working_gyro.vi"("Parâmetros Iniciais"=w286, "NXT/EV3"=w287) -> ("NXT/EV3 2"=w285:T7)  [unwired: 9 in]
                    n33 = call <vilib>:"EV3_Gyro_Angle.vi"("NXT/EV3"=w285, "Port (Port 1)"=w283) -> ("Degrees"=w282:sgl, "NXT/EV3"=w284:T7)  [unwired: 1 in]
                  }
                }
                n34 = call <vilib>:"Rotation.vi"("NXT/EV3"=w271, "Port (Port A)"=w276) -> ("Angle of Rotation"=w274:i32, "NXT/EV3"=w275:T7)  [unwired: 1 in]
              }
            }
            n35 = call <vilib>:"EV3_Ultrasonic_CM.vi"("NXT/EV3"=w184, "Port (Port 1)"=w164) -> ("Centimeters"=w183:sgl, "NXT/EV3"=w181:T7)  [unwired: 1 in]
            n36 = Greater Or Equal?(x=w183, y=sgl 8.5) -> (x >= y?=w174:bool)
            n37 = case shown="\"Front\"" w172 {
              tunnel: w181 -> [w190 w193 w201 w204]
              tunnel: [w190 w197 w200 w204] -> w163
              tunnel: [w188 w192 w199 w203] -> w171
              tunnel: w154 -> [_ w196 _ _]
              tunnel: w159 -> [_ w195 _ _]
              tunnel: w160 -> [_ w194 _ _]
              tunnel: [FALSE w192 w199 w203] -> w158
              tunnel: [w188 TRUE FALSE FALSE] -> w161
              frame "Nada" {
                w188 = FALSE
              }
              frame "Front" {
                w192 = FALSE
                n38 = call "front.vi"("Parâmetros Ini 2"=w194, "NXT/EV3"=w193, "Características Ini"=w195, "First Angle"=w196) -> ("NXT/EV3 2"=w197:T7)  [unwired: 7 in]
              }
              frame "Pega" {
                w199 = TRUE
                n39 = call "catch.vi"("NXT/EV3"=w201) -> ("NXT/EV3 2"=w200:T7)  [unwired: 10 in]
              }
              frame "Fim" {
                w203 = TRUE
              }
            }
            n40 = And(x=w171, y=w168) -> (x .and. y?=w170:bool)
            n41 = case shown="False" w173 {
              tunnel: [w210 enum16{"Nada", "Front", "Pega", "Fim"}."Nada" ("Movimentos \nStop")] -> w176
              tunnel: w172 -> [_ _]
              tunnel: w174 -> [w211 _]
              tunnel: w163 -> [w209 w232]
              tunnel: [w208 w232] -> w162
              tunnel: w161 -> [w207 _]
              frame False {
                n42 = case shown="False" w211 {
                  tunnel: [enum16{"Nada", "Front", "Pega", "Fim"}."Pega" ("Movimentos \nStop") enum16{"Nada", "Front", "Pega", "Fim"}."Front" ("Movimentos \nStop")] -> w210
                  tunnel: w209 -> [w214 w230]
                  tunnel: [w213 w230] -> w208
                  tunnel: w207 -> [w212 _]
                  frame False {
                    n43 = case shown="True" w212 {
                      tunnel: w214 -> [w216 w220]
                      tunnel: [w216 w218] -> w213
                      frame False {
                      }
                      frame True {
                        w217 = i8 0 ("Power/Speed 1")
                        n44 = xnode "Motors"() -> ("Motor"=w219:cluster{"Port":T8, "Port":T8})
                        n45 = xnode "Move Motors"("Power/Speed 2"=w217, "Power/Speed 1"=w217, "Motors"=w219, "NXT/EV3"=w220) -> ("NXT/EV3"=w218:T7)
                      }
                    }
                  }
                  frame True {
                  }
                }
              }
              frame True {
              }
            }
            n46 = case shown="True" w170 {
              selector: w170 -> [w249 _]
              tunnel: [w249 w250] -> w157
              tunnel: w162 -> [w248 w253]
              tunnel: w167 -> [_ w257]
              tunnel: [w248 w256] -> w179
              tunnel: w160 -> [_ w255]
              tunnel: w154 -> [_ w254]
              tunnel: w159 -> [_ w252]
              tunnel: [w247 w250] -> w155
              tunnel: w156 -> [w247 _]
              frame False {
              }
              frame True {
                n47 = call "backwards.vi"("Parâmetros Ini 2"=w255, "NXT/EV3"=w253, "Características Ini"=w252, "First Angle"=w254) -> ("NXT/EV3 2"=w251:T7)  [unwired: 7 in]
                n48 = xnode "Motors"() -> ("Motor"=w261:T8)
                n49 = call <vilib>:"Rotation.vi"("NXT/EV3"=w251, "Port (Port A)"=w261) -> ("Angle of Rotation"=w258:i32, "NXT/EV3"=w256:T7)  [unwired: 1 in]
                n50 = Subtract(x=w257, y=w258) -> (x-y=w259:i32)
                n51 = Less Or Equal?(x=w259, y=0) -> (x <= y?=w250:bool)
              }
            }
            n52 = case shown="True" w158 {
              tunnel: w176 -> [w205 _]
              tunnel: [w205 enum16{"Nada", "Front", "Pega", "Fim"}."Fim" ("Movimentos \nStop")] -> w175
              frame False {
              }
              frame True {
              }
            }
            n53 = case shown="True" w155 {
              selector: w155 -> [w235 _]
              tunnel: w180 -> [_ w240]
              tunnel: [w235 w237] -> w178
              tunnel: w179 -> [_ w239]
              tunnel: w160 -> [_ w238]
              tunnel: [TRUE FALSE] -> w169
              frame False {
              }
              frame True {
                n54 = case shown="False" w240 {
                  tunnel: w239 -> [w243 w246]
                  tunnel: w238 -> [w242 w245]
                  tunnel: [w241 w244] -> w237
                  frame False {
                    n55 = call "right.vi"("Parâmetros Ini 2"=w242, "NXT/EV3"=w243) -> ("x = y?"=w241:bool)  [unwired: 8 in, 1 out]
                  }
                  frame True {
                    n56 = call "left.vi"("Parâmetros Ini 2"=w245, "NXT/EV3"=w246) -> ("x = y?"=w244:bool)  [unwired: 8 in, 1 out]
                  }
                }
              }
            }
            n57 = Or(x=FALSE, y=w178) -> (x .or. y?=w165:bool)
          }
          frame "End" {
            n58 = call "working_gyro.vi"("Parâmetros Iniciais"=w301, "NXT/EV3"=w303) -> ("NXT/EV3 2"=w302:T7)  [unwired: 9 in]
            n59 = call "turn_back.vi"("Parâmetros Ini 2"=w301, "NXT/EV3"=w302, "First angle"=w310) -> ("x = y?"=w311:bool)  [unwired: 7 in]
          }
          frame "Intersection" {
            # "Com a flat sequence o robô realiza por etapas os movimentos na intersection, pois após virar para os lados ele deverá andar para\nfrente até encontrar branco. Quando encontrar branco o booleano muda para true ,permitindo mudança de estado."
            n60 = Unbundle By Name(w333) -> ("Colors and Directions"=w344:enum16{"Zero", "Right", "Front", "Left"}[])
            n61 = Bundle By Name(cluster=w317, "Old Color"=w342) -> (w343:T2)
            n62 = Index Array(array=w344, index=w342) -> (element=w345:enum16{"Zero", "Right", "Front", "Left"})
            n63 = local write "Características"(w343) -> ()
            n64 = case shown="True" w316 {
              tunnel: w315 -> [_ w350]
              tunnel: w314 -> [_ w349]
              tunnel: [FALSE w347] -> w313
              frame False {
              }
              frame True {
                n65 = call "identColor.vi"("Parâmetros Ini"=w349, "NXT/EV3"=w350) -> ("Collor"=w351:T3)  [unwired: 9 in]
                n66 = Equal?(x=w351, y=ColorSensorColors."White" ("Collor")) -> (x = y?=w348:bool)
                n67 = Not(x=w348) -> (.not. x?=w347:bool)
              }
            }
            n68 = case shown="True" w313 {
              tunnel: w315 -> [w416 w419]
              tunnel: [w416 w417] -> w341
              tunnel: w314 -> [_ w418]
              frame False {
              }
              frame True {
                n69 = call "turning_correction.vi"("Parâmetros Ini 2"=w418, "NXT/EV3"=w419) -> ("NXT/EV3 2"=w417:T7)  [unwired: 9 in]
              }
            }
            n70 = Not(x=w324) -> (.not. x?=w332:bool)
            n71 = case shown="True" w332 {
              tunnel: [FALSE w376] -> w330
              tunnel: w345 -> [_ w375]
              tunnel: w342 -> [_ w374]
              tunnel: w341 -> [w363 w373]
              tunnel: [FALSE w372] -> w336
              tunnel: [TRUE w371] -> w319
              tunnel: w314 -> [_ w370]
              tunnel: w333 -> [_ w369]
              tunnel: [w363 w368] -> w328
              tunnel: w325 -> [_ w367]
              frame False {
              }
              frame True {
                n72 = case shown="\"Zero\", Default" w375 {
                  tunnel: [FALSE FALSE w396 FALSE] -> w376
                  tunnel: w373 -> [w382 w388 w395 w404]
                  tunnel: w370 -> [_ _ w394 _]
                  tunnel: w370 -> [w381 w387 _ w403]
                  tunnel: w369 -> [_ _ w398 _]
                  tunnel: w374 -> [_ _ w393 _]
                  tunnel: [FALSE FALSE FALSE FALSE] -> w372
                  tunnel: [w378 w384 FALSE w400] -> w371
                  tunnel: [w377 w383 w390 w399] -> w368
                  tunnel: w367 -> [_ _ w389 _]
                  frame "Zero", Default {
                    n73 = call "right.vi"("Parâmetros Ini 2"=w381, "NXT/EV3"=w382) -> ("x = y?"=w378:bool, "NXT/EV3 2"=w377:T7)  [unwired: 8 in]
                  }
                  frame "Left" {
                    n74 = call "left.vi"("Parâmetros Ini 2"=w387, "NXT/EV3"=w388) -> ("x = y?"=w384:bool, "NXT/EV3 2"=w383:T7)  [unwired: 8 in]
                  }
                  frame "Front" {
                    n75 = call "front.vi"("Parâmetros Ini 2"=w394, "NXT/EV3"=w395, "Características Ini"=w398, "First Angle"=w389) -> ("NXT/EV3 2"=w390:T7)  [unwired: 7 in]
                    n76 = Equal?(x=w393, y=ColorSensorColors."White") -> (x = y?=w396:bool)
                  }
                  frame "Right" {
                    n77 = call "right.vi"("Parâmetros Ini 2"=w403, "NXT/EV3"=w404) -> ("x = y?"=w400:bool, "NXT/EV3 2"=w399:T7)  [unwired: 8 in]
                  }
                }
              }
            }
            n78 = And(x=w324, y=w322) -> (x .and. y?=w323:bool)
            n79 = case shown="True" w323 {
              tunnel: w328 -> [w354 w362]
              tunnel: [w354 w360] -> w327
              tunnel: w314 -> [_ w359]
              tunnel: [w355 w357] -> w326
              tunnel: w325 -> [w355 _]
              tunnel: [w353 TRUE] -> w320
              tunnel: w318 -> [w353 _]
              frame False {
              }
              frame True {
                n80 = call "working_gyro.vi"("Parâmetros Iniciais"=w359, "NXT/EV3"=w362) -> ("NXT/EV3 2"=w361:T7)  [unwired: 9 in]
                n81 = Unbundle By Name(w359) -> ("Gyro Port"=w358:T6)
                n82 = call <vilib>:"EV3_Gyro_Angle.vi"("NXT/EV3"=w361, "Port (Port 1)"=w358) -> ("Degrees"=w357:sgl, "NXT/EV3"=w360:T7)  [unwired: 1 in]
              }
            }
            n83 = case shown="True" w318 {
              tunnel: w314 -> [_ w411]
              tunnel: w333 -> [_ w407]
              tunnel: w327 -> [_ w415]
              tunnel: [FALSE w409] -> w329
              tunnel: w326 -> [_ w410]
              tunnel: [TRUE FALSE] -> w321
              tunnel: w317 -> [_ _]
              frame False {
              }
              frame True {
                n84 = call "front.vi"("Parâmetros Ini 2"=w411, "NXT/EV3"=w415, "Características Ini"=w407, "First Angle"=w410) -> ("NXT/EV3 2"=w412:T7)  [unwired: 7 in]
                n85 = call "identColor.vi"("Parâmetros Ini"=w411, "NXT/EV3"=w412) -> ("Collor"=w413:T3)  [unwired: 9 in]
                n86 = Equal?(x=w413, y=ColorSensorColors."White") -> (x = y?=w409:bool)
              }
            }
            n87 = Or(x=w330, y=w329) -> (x .or. y?=w331:bool)
          }
          frame "Empty" {
          }
        }
      }
    }
    "Enable" <- w44
    n88 = case shown="True" w44 {
      tunnel: [w444 FALSE ("Boolean")] -> w51
      tunnel: [w443 FALSE ("Boolean")] -> w50
      tunnel: [w442 w450] -> w49
      tunnel: w55 -> [w444 _]
      tunnel: w54 -> [w443 _]
      tunnel: w53 -> [w442 _]
      tunnel: w52 -> [w441 _]
      tunnel: [w441 w450] -> w48
      tunnel: [w440 enum16{"Nada", "Front", "Pega", "Fim"}."Nada" ("Movimentos \nStop")] -> w47
      tunnel: w46 -> [w440 _]
      frame False {
      }
      frame True {
        w450 = TRUE
        # "Resetando stop"
        n89 = local read "Booleanos e Contadores"() -> (w446:T1)
        n90 = Unbundle By Name(w446) -> ("Bonecos"=w448:dbl)
        n91 = Increment(x=w448) -> (x+1=w447:dbl)
        n92 = Bundle By Name(cluster=w446, "Bonecos"=w447) -> (w445:T1)
        n93 = local write "Booleanos e Contadores"(w445) -> ()
      }
    }
    "Boolean" <- w51
    "Boolean 2" <- w50
    "Boolean 3" <- w49
    "Boolean 4" <- w48
    n94 = case shown="True" w44 {
      tunnel: [w435 TRUE] -> w43
      tunnel: [w434 FALSE] -> w42
      tunnel: w30 -> [w435 _]
      tunnel: w35 -> [w434 _]
      tunnel: [w433 TRUE] -> w39
      tunnel: w38 -> [w433 _]
      tunnel: [w432 FALSE] -> w37
      tunnel: w36 -> [w432 _]
      frame False {
      }
      frame True {
      }
    }
  }
  n95 = call-poly <vilib>:"PolyDisplay.vi"("NXT/EV3"=w7) -> ()  [unwired: 3 in, 1 out]
  n96 = while {
    tunnel: w7 -> [w472]
    tunnel: w23 -> [w471]
    shift-right: [w453] -> _
    shift-left: "Características Iniciais" -> [w470]
    shift-right: [w457] -> _
    shift-left: "Booleanos e Contadores Iniciais" -> [w469]
    shift-right: [w454] -> _
    shift-left: ColorSensorColors."White" ("Detected Color") -> [w465]
    stop <- TRUE continue-if-true
    w461 = T10 2 items=["Enter button"=3, "Left button"=2, "Right button"=1, "Up Button"=4, "Down Button"=5] ("Button (Enter button)")
    # "Voltar caso dê pau em algum momento"
    # "Printar na tela a direção , estado e cor atual"
    # "State Machine"
    n97 = local read "Enable\nreforço SM"() -> (w467:bool)
    n98 = local read "Enable"() -> (w466:bool)
    n99 = Unbundle By Name(w470) -> ("Colors and Directions"=w475:enum16{"Zero", "Right", "Front", "Left"}[])
    n100 = call "identColor.vi"("Parâmetros Ini"=w471, "NXT/EV3"=w472) -> ("Collor"=w463:T3)  [unwired: 9 in]
    "Collor" <- w463
    "IdentifyCollor" <- w463
    n101 = Unbundle By Name(w470) -> ("CS"=w474:T9)
    n102 = local read "IdentifyCollor"() -> (w473:T3)
    n103 = And(x=w466, y=w467) -> (x .and. y?=w468:bool)
    n104 = Index Array(array=w475, index=w463) -> (element=w476:enum16{"Zero", "Right", "Front", "Left"})
    n105 = Unbundle By Name(w470) -> ("Old Color"=w464:T3)
    n106 = call "analysis.vi"("Collor"=w473, "CS 2"=w474, "Direction"=w476) -> ()  [unwired: 9 in]
    n107 = call "last_intersection_check.vi"("Last intersection color"=w465, "Old color"=w464, "Identify Color"=w463) -> ("Color 3"=w462:T3, "Color 2"=w455:T3)  [unwired: 7 in]
    n108 = case shown="True" w468 {
      selector: w468 -> [_ w508]
      tunnel: w462 -> [w504 w515]
      tunnel: w472 -> [_ w514]
      tunnel: [w504 w513] -> _
      tunnel: w471 -> [_ w512]
      tunnel: w470 -> [w503 w507]
      tunnel: [w503 w511] -> w459
      tunnel: w469 -> [w502 w510]
      tunnel: [w502 w509] -> w457
      frame False {
        n109 = local read "Enable"() -> (w501:bool)
        n110 = case shown="False" w501 {
          frame False {
            n111 = local write "Enable\nreforço SM"(TRUE ("Enable\nreforço SM")) -> ()
          }
          frame True {
          }
        }
      }
      frame True {
        n112 = Unbundle By Name(w507) -> ("CS"=w506:T9)
        n113 = case shown="\"Intersection\"" w506 {
          tunnel: w515 -> [w523 w529 w559 w580 w626 w675]
          tunnel: w514 -> [_ w530 _ _ w625 _]
          tunnel: [w523 w529 w559 w581 w624 w675] -> w513
          tunnel: w512 -> [_ w528 _ _ w623 _]
          tunnel: w512 -> [_ _ _ _ w620 _]
          tunnel: w507 -> [w522 w527 w561 w572 w619 w674]
          tunnel: [w520 w526 w560 w579 w618 w673] -> w511
          tunnel: w510 -> [w519 w525 w558 w576 w617 w672]
          tunnel: [w517 w525 w558 w575 w616 w671] -> w509
          tunnel: w508 -> [_ w524 _ _ _ _]
          frame "Delivery" {
            # "Manda o n de inter\n para o total"
            # "Booleano do contador\nde interseções"
            # "Enquanto não sabemos\ncomo controlar a quantidade\nde bonecos que já pegamos,\nvamos dizer que ele sempre\nvolta pra street para coletar mais bonecos"
            n114 = Unbundle By Name(w519) -> ("Intersections crossed"=w518:dbl)
            n115 = Bundle By Name(cluster=w519, "Intersections crossed total"=w518, "First End"=FALSE) -> (w517:T1)
            n116 = Bundle By Name(cluster=w522, "CS"=enum16{"Street", "Intersection", "End", "Stop"}."Street") -> (w520:T2)
          }
          frame "Stop" {
            n117 = disable-structure shown="Enabled" {
              disable-tunnel: w530 -> [w537 _]
              disable-tunnel: w528 -> [w536 _]
              disable-tunnel: w527 -> [w532 w550]
              disable-tunnel: [w531 w551] -> w526
              disable-tunnel: w524 -> [_ w549]
              frame Disabled {
                n118 = Unbundle By Name(w536) -> ("Sensor - Left"=w533:T6, "Sensor - Right"=w534:T6, "Distance to street"=w535:dbl)
                n119 = call <vilib>:"Sonar_cm.vi"("NXT/EV3"=w537, "Port (Port 4)"=w533) -> ("Distance (cm)"=w539:i16)  [unwired: 1 in, 1 out]
                n120 = call <vilib>:"Sonar_cm.vi"("NXT/EV3"=w537, "Port (Port 4)"=w534) -> ("Distance (cm)"=w538:i16)  [unwired: 1 in, 1 out]
                n121 = Greater Or Equal?(x=w539, y=w535) -> (x >= y?=w541:bool)
                n122 = Greater Or Equal?(x=w538, y=w535) -> (x >= y?=w542:bool)
                n123 = And(x=w541, y=w542) -> (x .and. y?=w540:bool)
                n124 = case shown="False" w540 {
                  tunnel: w532 -> [w544 w548]
                  tunnel: [w543 w546] -> w531
                  frame False {
                    n125 = Bundle By Name(cluster=w544, "CS"=enum16{"Street", "Intersection", "End", "Stop"}."Stop") -> (w543:T2)
                  }
                  frame True {
                    n126 = Bundle By Name(cluster=w548, "CS"=enum16{"Street", "Intersection", "End", "Stop"}."Street") -> (w546:T2)
                  }
                }
              }
              frame Enabled {
                n127 = case shown="False" w549 {
                  tunnel: [w552 w556] -> w551
                  tunnel: w550 -> [w553 w555]
                  frame False {
                    n128 = Bundle By Name(cluster=w553, "CS"=enum16{"Street", "Intersection", "End", "Stop"}."Stop") -> (w552:T2)
                  }
                  frame True {
                    n129 = Bundle By Name(cluster=w555, "CS"=enum16{"Street", "Intersection", "End", "Stop"}."Street") -> (w556:T2)
                  }
                }
              }
            }
          }
          frame "Square" {
            n130 = Equal?(x=w559, y=ColorSensorColors."Black") -> (x = y?=w562:bool)
            n131 = case shown="True" w562 {
              tunnel: w561 -> [w566 w570]
              tunnel: [w564 w569] -> w560
              frame False {
                n132 = Bundle By Name(cluster=w566, "CS"=T4."Square") -> (w564:T2)
              }
              frame True {
                n133 = Bundle By Name(cluster=w570, "CS"=T4."Delivery") -> (w569:T2)
                n134 = local write "Enable\nreforço SM"(FALSE) -> ()
              }
            }
          }
          frame "Intersection" {
            # "Se cor atual = cor antiga: passa\nbranco como cor atual."
            # "O Old Color vê qual foi a cor da última interseção. Se ela não estiver cadastrada em Colors and Directions, significa\nque seu valor é Zero."
            n135 = Unbundle By Name(w572) -> ("Colors and Directions"=w578:enum16{"Zero", "Right", "Front", "Left"}[], "Old Color"=w577:T3)
            n136 = Equal?(x=w580, y=w577) -> (x = y?=w582:bool)
            n137 = Index Array(array=w578, index=w577) -> (element=w583:enum16{"Zero", "Right", "Front", "Left"})
            n138 = case shown="False" w582 {
              tunnel: [w585 ColorSensorColors."White" ("Detected Color")] -> w581
              tunnel: w580 -> [w585 _]
              frame False {
              }
              frame True {
              }
            }
            n139 = Equal To 0?(x=w583) -> (x = 0?=w584:bool)
            n140 = Bundle By Name(cluster=w572, "CS"=T9."Street") -> (w571:T2)
            n141 = case shown="True" w584 {
              tunnel: w571 -> [w588 w597]
              tunnel: [w588 w596] -> w579
              tunnel: w576 -> [w590 w595]
              tunnel: [w589 w594] -> w575
              tunnel: [TRUE w592] -> w574
              frame False {
                # "Aqui ele já conhece a cor. Volta para Street e o \nBoolean volta a ser False."
                n142 = Bundle By Name(cluster=w590, "Correct"=FALSE) -> (w589:T1)
              }
              frame True {
                # "Testamos se o Boolean é True"
                n143 = Unbundle By Name(w595) -> ("Correct"=w593:bool)
                n144 = case shown="True" w593 {
                  tunnel: w597 -> [w599 w610]
                  tunnel: [w599 w613] -> w596
                  tunnel: w595 -> [w600 w607]
                  tunnel: [w601 w605] -> w594
                  tunnel: [w598 TRUE] -> w592
                  frame False {
                    w598 = TRUE
                    # "Volta para Street e o Boolean\nvira True; o robô ainda não\nacertou."
                    n145 = Bundle By Name(cluster=w600, "Correct"=w598) -> (w601:T1)
                  }
                  frame True {
                    # "Acertô, Mizeravi"
                    n146 = Unbundle By Name(w610) -> ("Colors and Directions"=w604:enum16{"Zero", "Right", "Front", "Left"}[], "Direction"=w609:enum16{"Zero", "Right", "Front", "Left"}, "Old Color"=w603:T3)
                    n147 = call "intersection_counter.vi"("Booleanos e Contadores Iniciais"=w607) -> ("Intersections crossed"=w606:dbl)  [unwired: 8 in]
                    n148 = Replace Array Subset(array=w604, new element=w609, index=w603) -> (w611:enum16{"Zero", "Right", "Front", "Left"}[])
                    n149 = Bundle By Name(cluster=w610, "Direction"=enum16{"Zero", "Right", "Front", "Left"}."Right", "Colors and Directions"=w611) -> (w613:T2)
                    n150 = Bundle By Name(cluster=w607, "Intersections crossed"=w606, "Correct"=TRUE) -> (w605:T1)
                  }
                }
              }
            }
            "Boolean 5" <- w574
          }
          frame "Street", Default {
            # "Se não for preto, ou é Intersection ou é Street."
            n151 = Not Equal?(x=w626, y=ColorSensorColors."Black" ("Detected Color")) -> (x != y?=w627:bool)
            n152 = Unbundle By Name(w623) -> ("Distance to street"=w615:dbl, "Sensor - Left"=w621:T6, "Sensor - Right"=w622:T6)
            n153 = case shown="True" w627 {
              tunnel: w626 -> [w636 w646]
              tunnel: w625 -> [_ w647]
              tunnel: [w636 w646] -> w624
              tunnel: w622 -> [_ w645]
              tunnel: w621 -> [_ w644]
              tunnel: w620 -> [_ w643]
              tunnel: w619 -> [w633 w642]
              tunnel: [w634 w641] -> w618
              tunnel: w617 -> [w630 w640]
              tunnel: [w630 w639] -> w616
              tunnel: w615 -> [_ w638]
              tunnel: [FALSE w637] -> w614
              frame False {
                # "Nesse caso, ele chegou numa dead-end; vai para o estado End\ne adiciona um no contador."
                n154 = Unbundle By Name(w633) -> ("Direction"=w632:enum16{"Zero", "Right", "Front", "Left"})
                n155 = Increment(x=w632) -> (x+1=w631:enum16{"Zero", "Right", "Front", "Left"})
                n156 = Bundle By Name(cluster=w633, "CS"=enum16{"Street", "Intersection", "End"}."End", "Direction"=w631) -> (w634:T2)
              }
              frame True {
                # "Se não for branco, ou é Intersection ou é Square"
                n157 = Not Equal?(x=w646, y=ColorSensorColors."White" ("Detected Color")) -> (x != y?=w648:bool)
                n158 = case shown="True" w648 {
                  tunnel: w647 -> [w651 w667]
                  tunnel: w645 -> [w659 _]
                  tunnel: w644 -> [w658 _]
                  tunnel: w643 -> [_ w664]
                  tunnel: w642 -> [w657 w666]
                  tunnel: [w656 w665] -> w641
                  tunnel: w640 -> [w655 w663]
                  tunnel: [w654 w663] -> w639
                  tunnel: w638 -> [w652 _]
                  tunnel: [w650 w662] -> w637
                  frame False {
                    # "Ou ele vai para Stop ou continua em Street"
                    n159 = call <vilib>:"EV3_Ultrasonic_CM.vi"("NXT/EV3"=w651, "Port (Port 1)"=w658) -> ("Centimeters"=w661:sgl)  [unwired: 1 in, 1 out]
                    n160 = call <vilib>:"EV3_Ultrasonic_CM.vi"("NXT/EV3"=w651, "Port (Port 1)"=w659) -> ("Centimeters"=w660:sgl)  [unwired: 1 in, 1 out]
                    n161 = call "toStop.vi"("Left"=w660, "Distance to street"=w652, "Booleanos e Contadores Iniciais IN"=w655, "Características in"=w657, "Right"=w661) -> ("Boolean"=→"Direction Bool":bool, "Booleanos e Contadores Iniciais OUT"=w654:T1, "Características out"=w656:T11, "Enable 2"=w650:bool)  [unwired: 7 in]
                  }
                  frame True {
                    n162 = call "squareOrIntersection.vi"("Características in"=w666, "Parâmetros Ini 2"=w664, "NXT/EV3"=w667) -> ("Características out"=w665:T11, "Boolean"=w662:bool)  [unwired: 5 in]
                  }
                }
              }
            }
            "Enable\nreforço SM" <- w614
          }
          frame "End" {
            # "Depois de um End, ele sempre volta para Street, e o Boolean vira False"
            n163 = Bundle By Name(cluster=w674, "CS"=enum16{"Street", "Intersection", "End"}."Street") -> (w673:T2)
            n164 = Bundle By Name(cluster=w672, "Correct"=FALSE) -> (w671:T1)
            n165 = call "analysis.vi"("CS 2"=T4."End") -> ()  [unwired: 11 in]
          }
        }
      }
    }
    n166 = call-poly <vilib>:"PolySensor.vi"("Button (Enter button)"=w461) -> ("Yes/No"=w460:bool, "NXT/EV3"=w458:T7)  [unwired: 2 in]
    n167 = case shown="False" w460 {
      tunnel: w459 -> [w480 _]
      tunnel: [w480 T2 {"Colors and Directions"=[enum."Zero", enum."Zero", enum."Zero", enum."Zero", enum."Zero", enum."Zero"], "Direction"=enum."Right", "CS"=enum."Street", "Old Color"=enum."White"} ("Características Iniciais")] -> w453
      tunnel: w458 -> [_ w491]
      tunnel: w457 -> [w479 _]
      tunnel: [w479 T1 {"Correct"=FALSE, "Enable State change"=TRUE, "First End"=FALSE, "Intersections crossed"=0.0, "Intersections crossed total"=0.0, "Bonecos"=0.0} ("Booleanos e Contadores Iniciais")] -> w456
      tunnel: w455 -> [w478 _]
      tunnel: [w478 ColorSensorColors."White" ("Old Color")] -> w454
      frame False {
      }
      frame True {
        w484 = FALSE
        w485 = TRUE
        w493 = T10 4 items=["Enter button"=3, "Left button"=2, "Right button"=1, "Up Button"=4, "Down Button"=5] ("Button (Enter button)")
        n168 = xnode "Motors"() -> ("Motor"=w492:cluster{"Port":T8, "Port":T8})
        n169 = xnode "Stop Motors"("Motors"=w492, "NXT/EV3"=w491) -> ("NXT/EV3"=w490:T7)
        n170 = local write "Boolean 3"(w484) -> ()
        n171 = local write "Boolean 4"(w484) -> ()
        n172 = local write "Boolean 2"(w485) -> ()
        n173 = local read "Características"() -> (w483:T2)
        n174 = local write "Boolean"(w485) -> ()
        n175 = Bundle By Name(cluster=w483, "CS"=T9."Empty") -> (w482:T2)
        n176 = local write "Enable\nreforço SM"(TRUE) -> ()
        n177 = call-poly <vilib>:"PolyWait.vi"("NXT/EV3"=w490, "Button (Enter button)"=w493) -> ()  [unwired: 2 in, 1 out]
        n178 = local write "Características"(w482) -> ()
      }
    }
    "Características" <- w453
    "Booleanos e Contadores" <- w456
    n179 = disable-structure shown="Disabled" {
      frame Disabled {
        n180 = Wait (ms)(milliseconds to wait=u32 600) -> ()  [unwired: 1 out]
      }
      frame Enabled {
      }
    }
  }
